vi "Teleop.vi"(10 "Match Info":T1={"Autonomous Elapsed Seconds"=0.0, "TeleOp Elapsed Seconds"=0.0, "Disabled Elapsed Seconds"=0.0, "Visited Autonomous"=FALSE, "Visited TeleOp"=FALSE, "Visited Disabled"=FALSE, "Autonomous Settings"={"Autonomous Style"=enum."Independent", "VI Refnum"=refnum}}, 11 "Call Context":T2) -> ()   [LabVIEW 2015]
doc: "This VI is called for each TeleOp packet received from the DS where the robot is not disabled. It is often used to read from the joysticks and update I/O or to update setpoints for timed control loops. It should complete and return within 20 milliseconds or it may miss DS packets."
uses:
  <vilib>/Rock Robotics/WPI/DriverStation/WPI_DriverStationDerivedRobotMode.ctl
  <vilib>/Rock Robotics/WPI/DriverStation/WPI_DriverStationMatch Info.ctl
  <vilib>/Rock Robotics/WPI/Solenoid/WPI_SolenoidValue.ctl
  <vilib>/Rock Robotics/WPI/Relay/WPI_RelayValue.ctl
  Robot Global Data.vi
  <vilib>/Rock Robotics/WPI/Joystick/WPI_JoystickGetSetRefNum.vi
  <vilib>/Rock Robotics/WPI/RobotDrive/WPI_RobotDriveGetSetRefNum.vi
  <vilib>/Rock Robotics/WPI/RobotDrive/WPI_RobotDriveArcadeDrive_Standard(NoSaturation).vi
  <vilib>/Rock Robotics/WPI/Solenoid/WPI_SolenoidSetEnum.vi
panel:
  out "Numeric 1":dbl(slide) scale=0.0..100.0
  out "Boolean 2":bool
  out "Boolean 1":bool
  # "display DB vars here"
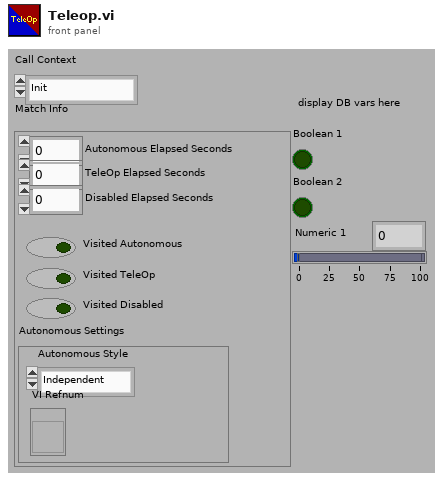
[diagram p1: front panel]
types:
  T1 = typedef "WPI_DriverStationMatch Info.ctl" = cluster{"Autonomous Elapsed Seconds":dbl, "TeleOp Elapsed Seconds":dbl, "Disabled Elapsed Seconds":dbl, "Visited Autonomous":bool, "Visited TeleOp":bool, "Visited Disabled":bool, "Autonomous Settings":cluster{"Autonomous Style":enum16{"Iterative", "Independent"}, "VI Refnum":refnum<vi>}}
  T2 = typedef "WPI_DriverStationDerivedRobotMode.ctl" = enum16{"Init", "Execute", "Stop"}
  T3 = typedef "WPI_JoystickDevRef.ctl" = cluster{"Device":T4}
  T4 = typedef "WPI_JoystickDeviceEnum.ctl" = enum16{"USB 0", "USB 1", "USB 2", "USB 3", "USB 4", "USB 5"}
  T5 = cluster{"axis 1 (x)":dbl, "axis 2 (y)":dbl, "axis 3 (throttle)":dbl, "axis 4":dbl, "axis 5":dbl, "axis 6":dbl}
  T6 = cluster{"Button 1":bool, "Button 2":bool, "Button 3":bool, "Button 4":bool, "Button 5":bool, "Button 6":bool, "Button 7":bool, "Button 8":bool, "Button 9":bool, "Button 10":bool, "Button 11":bool, "Button 12":bool}
  T7 = typedef "WPI_PWMDeviceRef.ctl" = cluster{"DeviceStatus":errorcluster, "Digital Module":T8, "PWM Channel":T9}
  T8 = typedef "FPGA_TypedefDigitalModule.ctl" = enum16{"Digital Module 1", "Digital Module 2"}
  T9 = typedef "FPGA_DIOPWMChannel.ctl" = enum8{"PWM 1", "PWM 2", "PWM 3", "PWM 4", "PWM 5", "PWM 6", "PWM 7", "PWM 8", "PWM 9", "PWM 10", "Invalid"}
  T10 = typedef "WPI_DigitalOutputDevRef.ctl" = cluster{"Digital Module":T8, "DIO Channel":T11, "DevStatus":errorcluster}
  T11 = typedef "FPGA_DIOChannel.ctl" = enum8{"DIO 1", "DIO 2", "DIO 3", "DIO 4", "DIO 5", "DIO 6", "DIO 7", "DIO 8", "DIO 9", "DIO 10", "DIO 11", "DIO 12", "DIO 13", "DIO 14", "Invalid"}
  T12 = typedef "WPI_RobotDriveDevRef.ctl" = cluster{"DevStatus":errorcluster, "Motors[]":T13[], "Square Inputs":bool, "Max Output":dbl}
  T13 = typedef "WPI_MotorControlDeviceRef.ctl" = cluster{"DeviceStatus":errorcluster, "Type":enum16{"PWM", "CAN"}, "PWM":cluster{"Digital Module":T8, "PWM Channel":T9, "DeadBand":T14}, "CAN":cluster{"Device Number":u8, "Control Mode":T15, "Semaphore":T16, "Max Vout":dbl}, "Invert":bool, "TransformRef":T17, "InvTransformRef":T17}
  T14 = typedef "WPI_PWMDeadband.ctl" = cluster{"Name":string, "maxPositivePwm":i32, "minPositivePwm":i32, "centerPwm":i32, "maxNegativePwm":i32, "minNegativePwm":i32, "angularRange":u16}
  T15 = typedef "WPI_CANJaguar_ControlMode.ctl" = enum8{"Percent VBus", "Current", "Speed", "Position", "Voltage"}
  T16 = typedef "Semaphore RefNum" = refnum<k1>
  T17 = typedef "WPI_PWMTransform_ConPane.ctl" = refnum<vi>
  T18 = typedef "WPI_SolenoidValue.ctl" = enum16{"Off", "On", "Forward", "Reverse"}
  T19 = typedef "WPI_RelayValue.ctl" = enum16{"Off", "On", "Forward", "Reverse"}
  T20 = typedef "WPI_RelayDevRef.ctl" = cluster{"DevStatus":errorcluster, "Relay Channel":T21, "Digital Module":T8, "Relay Direction":T22}
  T21 = typedef "FPGA_DIORelayChannel.ctl" = enum8{"Relay 1", "Relay 2", "Relay 3", "Relay 4", "Relay 5", "Relay 6", "Relay 7", "Relay 8", "Invalid"}
  T22 = typedef "WPI_RelayDirection.ctl" = enum16{"Both directions", "Forward only", "Reverse only"}
  T23 = typedef "WPI_SolenoidDevRef.ctl" = cluster{"DevStatus":errorcluster, "Solenoid Module":T24, "Forward Solenoid Channel":T25, "Reverse Solenoid Channel":T25}
  T24 = typedef "FPGA_TypedefSolenoidModule.ctl" = enum16{"Solenoid Module 1", "Solenoid Module 2"}
  T25 = typedef "WPI_SolenoidChannel.ctl" = enum8{"Solenoid 1", "Solenoid 2", "Solenoid 3", "Solenoid 4", "Solenoid 5", "Solenoid 6", "Solenoid 7", "Solenoid 8", "Invalid"}
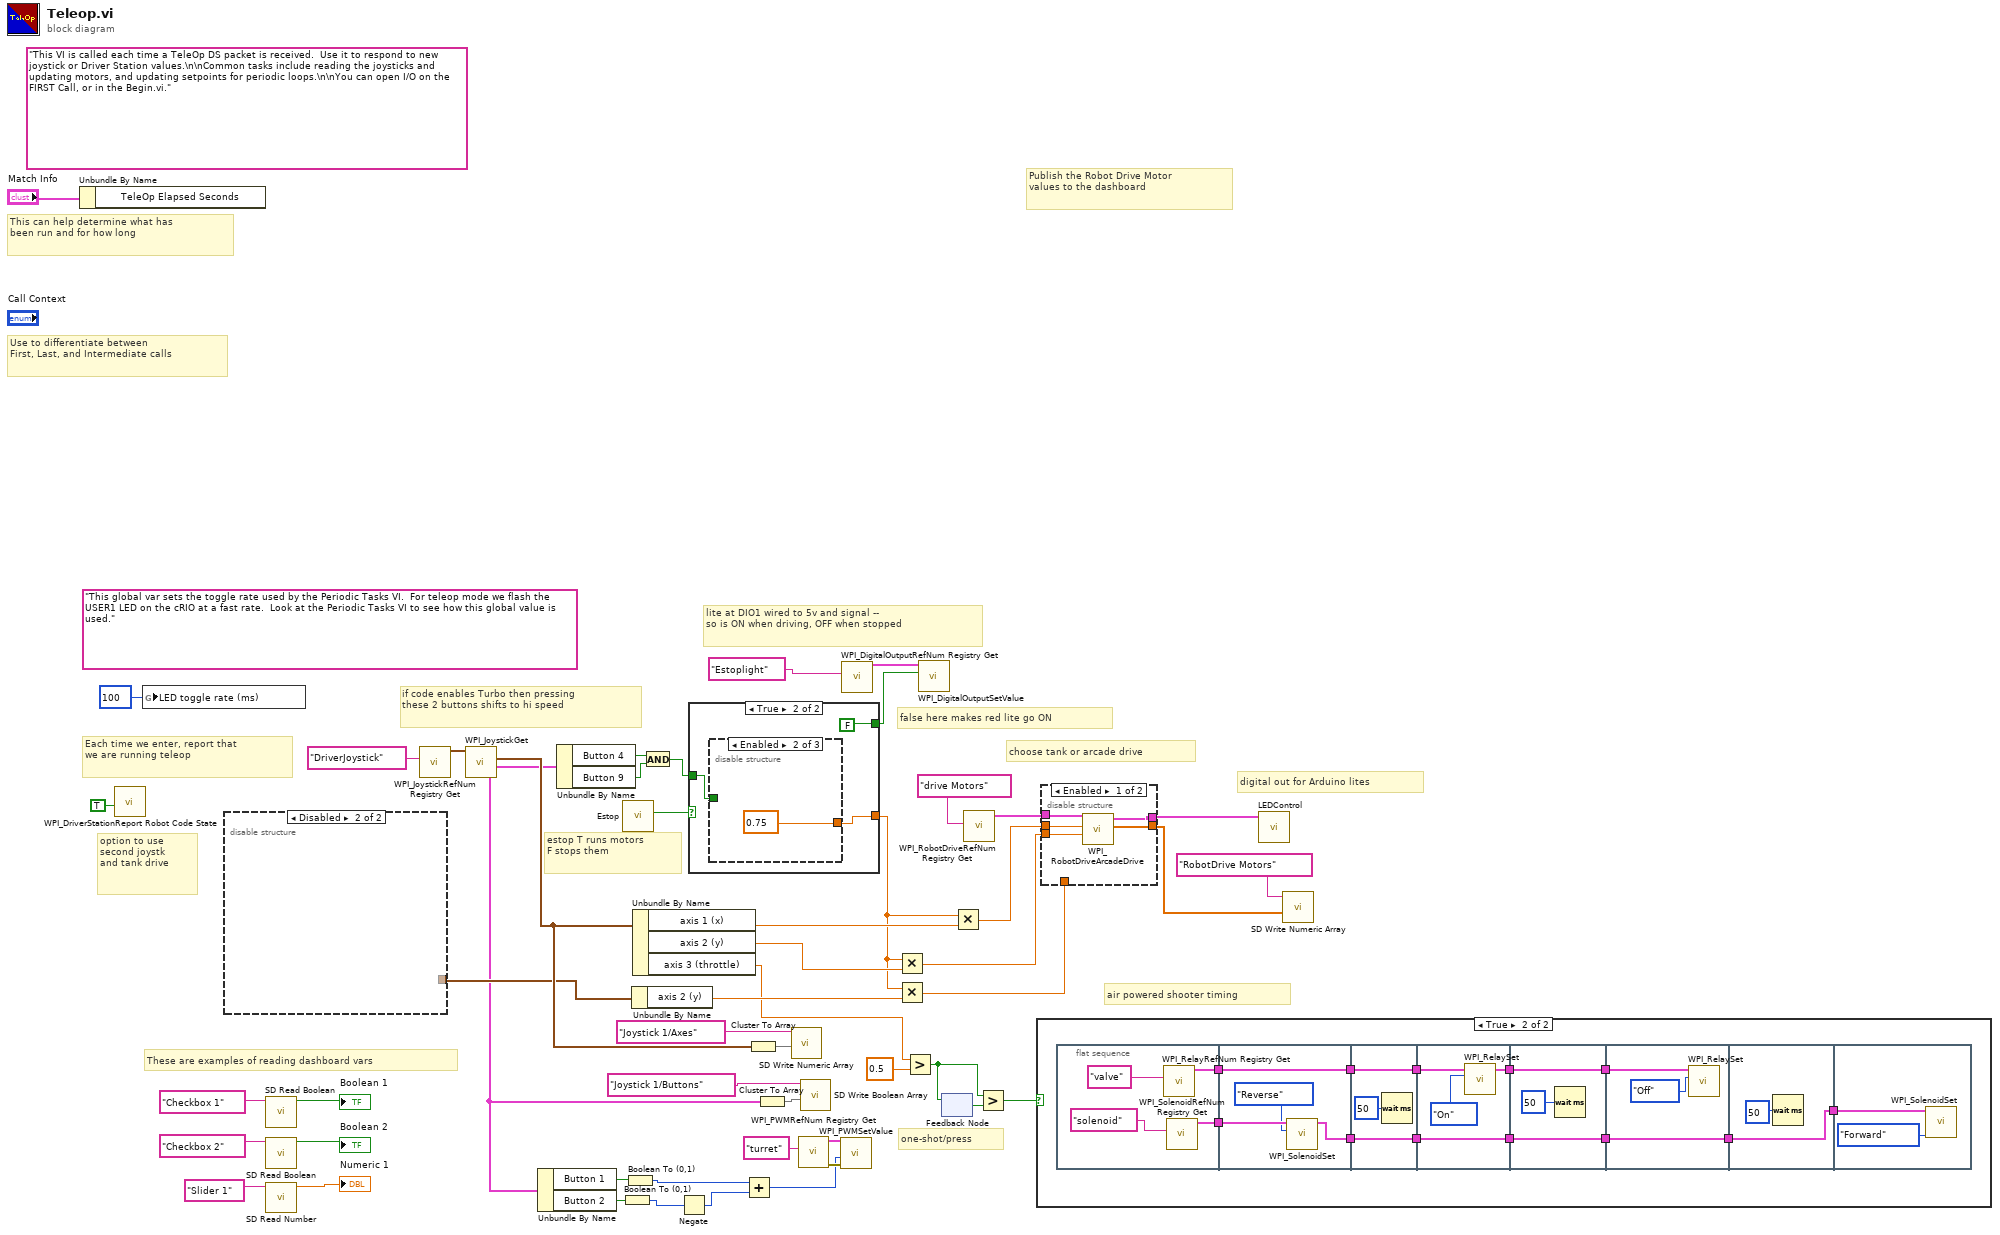
[diagram p0: block diagram]
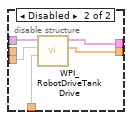
[diagram p3: hidden frame]
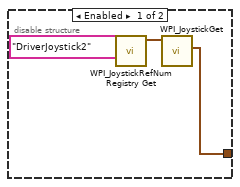
[diagram p4: hidden frame]
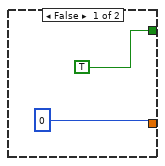
[diagram p5: hidden frame]
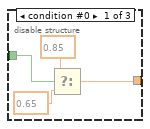
[diagram p6: hidden frame]
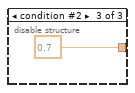
[diagram p7: hidden frame]
diagram:
  (unwired) "This global var sets the toggle rate used by the Periodic Tasks VI.  For teleop mode we flash the USER1 LED on the cRIO at a fast rate.  Look at the Periodic Tasks VI to see how this global value is used."
  (unwired) "This VI is called each time a TeleOp DS packet is received.  Use it to respond to new joystick or Driver Station values.\n\nCommon tasks include reading the joysticks and updating motors, and updating setpoints for periodic loops.\n\nYou can open I/O on the FIRST Call, or in the Begin.vi."
  # "air powered shooter timing"
  # "false here makes red lite go ON"
  # "option to use\nsecond joystk\nand tank drive"
  # "one-shot/press"
  # "estop T runs motors\nF stops them"
  # "if code enables Turbo then pressing\nthese 2 buttons shifts to hi speed"
  # "lite at DIO1 wired to 5v and signal --\nso is ON when driving, OFF when stopped"
  # "choose tank or arcade drive"
  # "digital out for Arduino lites"
  # "These are examples of reading dashboard vars"
  # "Publish the Robot Drive Motor\nvalues to the dashboard"
  # "Each time we enter, report that\nwe are running teleop"
  # "Use to differentiate between\nFirst, Last, and Intermediate calls"
  # "This can help determine what has\nbeen run and for how long"
  n1 = Unbundle By Name("Match Info") -> ()  [unwired: 1 out]
  n2 = call <vilib>:"WPI_DriverStationReport Robot Code State.vi"("TeleOp"=TRUE ("Autonomous")) -> ()  [unwired: 10 in, 1 out]
  n3 = global write "Robot Global Data.vi" "LED toggle rate (ms)"(u32 100 ("LED ms toggle rate")) -> ()
  n4 = disable-structure shown="Disabled" {
    disable-tunnel: [w52 _] -> w21
    frame Enabled {
      n5 = call <vilib>:"WPI_JoystickRefNum Registry Get.vi"("refnum name"="DriverJoystick2") -> ("JoystickDevRef"=w53:T3)  [unwired: 9 in, 1 out]
      n6 = call <vilib>:"WPI_JoystickGet.vi"("JoystickDevRef"=w53) -> ("Axes"=w52:T5)  [unwired: 4 in, 2 out]
    }
    frame Disabled {
    }
  }
  n7 = call <vilib>:"SD Read Boolean.vi"("Name"="Checkbox 1" ("refnum name")) -> ("Boolean"=→"Boolean 1":bool)  [unwired: 8 in, 2 out]
  n8 = call <vilib>:"SD Read Boolean.vi"("Name"="Checkbox 2" ("refnum name")) -> ("Boolean"=→"Boolean 2":bool)  [unwired: 8 in, 2 out]
  n9 = call <vilib>:"SD Read Number.vi"("Name"="Slider 1" ("refnum name")) -> ("Numeric"=→"Numeric 1":dbl)  [unwired: 8 in, 2 out]
  n10 = call <vilib>:"WPI_JoystickRefNum Registry Get.vi"("refnum name"="DriverJoystick") -> ("JoystickDevRef"=w39:T3)  [unwired: 9 in, 1 out]
  n11 = call <vilib>:"WPI_JoystickGet.vi"("JoystickDevRef"=w39) -> ("Buttons"=w15:T6, "Axes"=w23:T5)  [unwired: 4 in, 1 out]
  n12 = Unbundle By Name(w15) -> ("Button 1"=w14:bool, "Button 2"=w13:bool)
  n13 = Unbundle By Name(w15) -> ("Button 4"=w37:bool, "Button 9"=w36:bool)
  n14 = Boolean To (0,1)(Boolean=w13) -> (0, 1=w11:i16)
  n15 = call "Estop.vi"() -> ("Estop?"=w38:bool)  [unwired: 11 in]
  n16 = Boolean To (0,1)(Boolean=w14) -> (0, 1=w12:i16)
  n17 = Unbundle By Name(w21) -> ("axis 2 (y)"=w17:dbl)
  n18 = Unbundle By Name(w23) -> ("axis 1 (x)"=w34:dbl, "axis 2 (y)"=w20:dbl, "axis 3 (throttle)"=w5:dbl)
  n19 = And(x=w37, y=w36) -> (x .and. y?=w35:bool)
  n20 = Negate(x=w11) -> (-x=w10:i16)
  n21 = case shown="True" w38 {
    tunnel: w35 -> [_ w59]
    tunnel: [0 w58] -> w18
    tunnel: [TRUE FALSE] -> w30
    frame False {
    }
    frame True {
      n22 = disable-structure shown="Enabled" {
        disable-tunnel: w59 -> [w63 _ _]
        disable-tunnel: [w60 0.75 ("t") 0.7 ("t")] -> w58
        frame condition #0 {
          n23 = Select(t=0.85, s=w63, f=0.65) -> (s? t:f=w60:dbl)
        }
        frame condition #1 (active) {
        }
        frame condition #2 {
        }
      }
    }
  }
  n24 = Add(x=w12, y=w10) -> (x+y=w6:i16)
  n25 = Cluster To Array(cluster=w23) -> (array=w26:dbl[])
  n26 = Cluster To Array(cluster=w15) -> (array=w27:bool[])
  n27 = call <vilib>:"SD Write Numeric Array.vi"("Numeric Array"=w26, "Name"="Joystick 1/Axes") -> ()  [unwired: 8 in, 2 out]
  n28 = call <vilib>:"WPI_PWMRefNum Registry Get.vi"("refnum name"="turret") -> ("error out"=w8:errorcluster, "PWMDeviceRef"=w7:T7)  [unwired: 9 in]
  n29 = call <vilib>:"SD Write Boolean Array.vi"("Boolean Array"=w27, "Name"="Joystick 1/Buttons") -> ()  [unwired: 8 in, 2 out]
  n30 = call <vilib>:"WPI_PWMSetValue.vi"("error in (no error)"=w8, "Value"=w6, "PWMDeviceRef"=w7) -> ()  [unwired: 7 in, 2 out]
  n31 = call <vilib>:"WPI_DigitalOutputRefNum Registry Get.vi"("refnum name"="Estoplight") -> ("DigitalOutputDevRef"=w31:T10)  [unwired: 9 in, 1 out]
  n32 = Multiply(x=w18, y=w20) -> (x*y=w19:dbl)
  n33 = Multiply(x=w18, y=w17) -> (x*y=w16:dbl)
  n34 = Greater?(x=w5, y=0.5) -> (0:w2:bool)
  n35 = call <vilib>:"WPI_DigitalOutputSetValue.vi"("Value"=w30, "DigitalOutputDevRef"=w31) -> ()  [unwired: 8 in, 2 out]
  n36 = feedback-in #1(w2) -> ()
  n37 = feedback #1() -> (w3:bool)  [unwired: 1 in]
  n38 = Multiply(x=w18, y=w34) -> (x*y=w33:dbl)
  n39 = call <vilib>:"WPI_RobotDriveRefNum Registry Get.vi"("refnum name"="drive Motors") -> ("RobotDriveDevRef"=w41:T12)  [unwired: 9 in, 1 out]
  n40 = Greater?(x=w2, y=w3) -> (0:w1:bool)
  n41 = case shown="True" w1 {
    frame False {
    }
    frame True {
      n42 = flat-sequence {
        tunnel: [w79] -> w77
        tunnel: [w78] -> w76
        tunnel: w77 -> [w85]
        tunnel: [w83] -> w75
        tunnel: w76 -> [w83]
        tunnel: [w82] -> w67
        tunnel: w75 -> [w88]
        tunnel: [w88] -> w74
        tunnel: [w86] -> w68
        tunnel: w67 -> [w86]
        tunnel: w74 -> [w92]
        tunnel: [w90] -> w73
        tunnel: [w89] -> w69
        tunnel: w68 -> [w89]
        tunnel: w73 -> [w94]
        tunnel: [w94] -> w72
        tunnel: [w93] -> w70
        tunnel: w69 -> [w93]
        tunnel: w72 -> [w97]
        tunnel: [w96] -> w71
        tunnel: w70 -> [w96]
        tunnel: w71 -> [w99]
        tunnel: [w99] -> w66
        tunnel: w66 -> [w101]
        frame #0 {
          n43 = call <vilib>:"WPI_RelayRefNum Registry Get.vi"("refnum name"="valve") -> ("RelayDevRef"=w78:T20)  [unwired: 9 in, 1 out]
          n44 = call <vilib>:"WPI_SolenoidRefNum Registry Get.vi"("refnum name"="solenoid") -> ("SolenoidDevRef"=w79:T23)  [unwired: 9 in, 1 out]
        }
        frame #1 {
          n45 = call-poly <vilib>:"WPI_SolenoidSet.vi"("Value"=WPI_SolenoidValue."Reverse", "SolenoidDevRef"=w85) -> ("SolenoidDevRef"=w82:T23)  [unwired: 8 in, 1 out]
        }
        frame #2 {
          n46 = Wait (ms)(milliseconds to wait=u32 50) -> ()  [unwired: 1 out]
        }
        frame #3 {
          n47 = call <vilib>:"WPI_RelaySet.vi"("RelayValue"=WPI_RelayValue."On", "RelayDevRef"=w92) -> ("RelayDevRef"=w90:T20)  [unwired: 8 in, 1 out]
        }
        frame #4 {
          n48 = Wait (ms)(milliseconds to wait=u32 50) -> ()  [unwired: 1 out]
        }
        frame #5 {
          n49 = call <vilib>:"WPI_RelaySet.vi"("RelayValue"=WPI_RelayValue."Off", "RelayDevRef"=w97) -> ()  [unwired: 8 in, 2 out]
        }
        frame #6 {
          n50 = Wait (ms)(milliseconds to wait=u32 50) -> ()  [unwired: 1 out]
        }
        frame #7 {
          n51 = call-poly <vilib>:"WPI_SolenoidSet.vi"("Value"=WPI_SolenoidValue."Forward", "SolenoidDevRef"=w101) -> ()  [unwired: 8 in, 2 out]
        }
      }
    }
  }
  n52 = disable-structure shown="Enabled" {
    disable-tunnel: w41 -> [w107 w110]
    disable-tunnel: w33 -> [w106 _]
    disable-tunnel: w19 -> [w105 w109]
    disable-tunnel: [w104 w112] -> w24
    disable-tunnel: [w103 w111] -> w22
    disable-tunnel: w16 -> [_ w108]
    frame Enabled {
      n53 = call-poly <vilib>:"WPI_RobotDriveArcadeDrive.vi"("Y axis value"=w105, "X axis value"=w106, "RobotDriveDevRef"=w107) -> ("Motor Values"=w104:dbl[], "RobotDriveDevRef"=w103:T12)  [unwired: 6 in, 1 out]
    }
    frame Disabled {
      n54 = call <vilib>:"WPI_RobotDriveTankDrive.vi"("Right axis value"=w108, "Left axis value"=w109, "RobotDriveDevRef"=w110) -> ("Motor Values"=w112:dbl[], "RobotDriveDevRef"=w111:T12)  [unwired: 6 in, 1 out]
    }
  }
  n55 = call "LEDControl.vi"("RobotDriveDevRef 2"=w22) -> ()  [unwired: 11 in]
  n56 = call <vilib>:"SD Write Numeric Array.vi"("Numeric Array"=w24, "Name"="RobotDrive Motors") -> ()  [unwired: 8 in, 2 out]
